vi "single_shot_TRIG1.vi"(3 "error in (no error)":errorcluster, 5 "VISA resource name":refnum<visa-resource-name>) -> (0 "error out":errorcluster, 2 "VISA resource name 2":refnum<visa-resource-name>)   [LabVIEW 2012]
doc: "activates a single trigger"
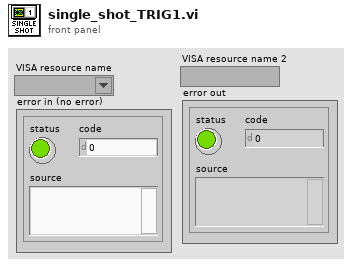
[diagram p1: front panel]
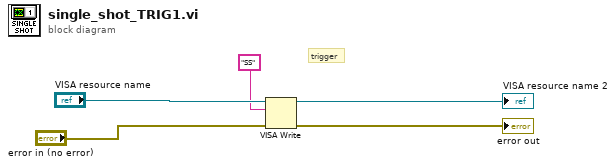
[diagram p0: block diagram]
diagram:
  # "trigger"
  n1 = VISA Write(VISA resource name="VISA resource name", write buffer="SS" ("command"), error in (no error)="error in (no error)") -> (VISA resource name out=→"VISA resource name 2":refnum<visa-resource-name>, error out=→"error out":errorcluster)  [unwired: 1 out]
